vi "Measure Digital Pulse Width.vi"   [LabVIEW 2017, in "NI_Robotics_FPGA Utilities.lvlib"]
uses:
  <vilib>/robotics/Utilities/FPGA Utilities/NI_Robotics_FPGA Utilities.lvlib
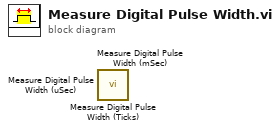
[diagram p0: block diagram]
diagram:
  n1 = call <vilib>:"Measure Digital Pulse Width (Ticks).vi"() -> ()  [unwired: 10 in, 2 out]
  n2 = call <vilib>:"Measure Digital Pulse Width (mSec).vi"() -> ()  [unwired: 10 in, 2 out]
  n3 = call <vilib>:"Measure Digital Pulse Width (uSec).vi"() -> ()  [unwired: 10 in, 2 out]
